vi "Run FGV Tests for String.vi"(2 "DELETE VI Reference":refnum<vi>, 3 "GET VI Reference":refnum<vi>, 4 "PUT VI Reference":refnum<vi>) -> (0 "Reason":string, 1 "Success":bool)   [LabVIEW 2013]
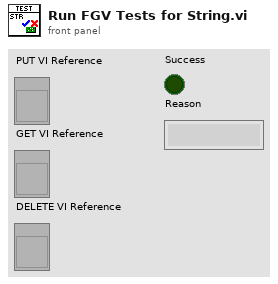
[diagram p1: front panel]
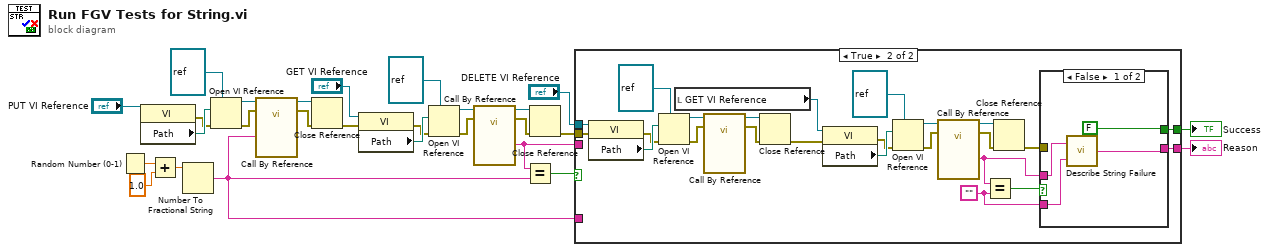
[diagram p0: block diagram]
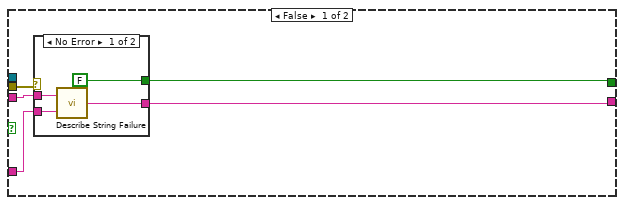
[diagram p2: hidden frame]
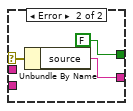
[diagram p3: hidden frame]
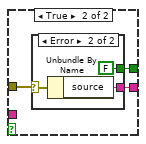
[diagram p4: hidden frame]
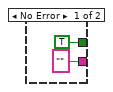
[diagram p5: hidden frame]
diagram:
  n1 = Random Number (0-1)() -> (number: 0 to 1=w12:dbl)
  n2 = property class="VI"(reference="PUT VI Reference") -> (error out=w5:errorcluster, "Path"=w18:path)  [unwired: 1 in, 1 out]
  n3 = Add(x=w12, y=1.0) -> (x+y=w2:dbl)
  n4 = Number To Fractional String(number=w2) -> (F-format string=w1:string)  [unwired: 3 in]
  n5 = Open VI Reference(type specifier VI Refnum (for type only)=refnum<vi> refnum, vi path=w18, error in (no error)=w5) -> (vi reference=w17:refnum<vi>, error out=w16:errorcluster)  [unwired: 3 in]
  n6 = call-by-ref "?"(reference=w17, error in=w16, "Division Input Channel"=w1) -> (reference out=w15:refnum<vi>, error out=w14:errorcluster)
  n7 = Close Reference(reference=w15, error in (no error)=w14) -> (error out=w10:errorcluster)
  n8 = property class="VI"(reference="GET VI Reference", error in=w10) -> (error out=w6:errorcluster, "Path"=w23:path)  [unwired: 1 out]
  n9 = Open VI Reference(type specifier VI Refnum (for type only)=refnum<vi> refnum, vi path=w23, error in (no error)=w6) -> (vi reference=w24:refnum<vi>, error out=w25:errorcluster)  [unwired: 3 in]
  n10 = call-by-ref "?"(reference=w24, error in=w25) -> (reference out=w26:refnum<vi>, error out=w27:errorcluster, "Division Input Channel"=w7:string)
  n11 = Equal?(x=w7, y=w1) -> (x = y?=w8:bool)
  n12 = Close Reference(reference=w26, error in (no error)=w27) -> (error out=w9:errorcluster)
  n13 = case shown="True" w8 {
    tunnel: "DELETE VI Reference" -> [_ w57]
    tunnel: w9 -> [w28 w56]
    tunnel: w1 -> [w31 _]
    tunnel: w7 -> [w32 _]
    tunnel: [w30 w42] -> w4
    tunnel: [w29 w41] -> w3
    frame False {
      n14 = case shown="No Error" w28 {
        selector: w28 -> [_ w39]
        tunnel: w32 -> [w36 _]
        tunnel: w31 -> [w35 _]
        tunnel: [FALSE FALSE] -> w30
        tunnel: [w33 w37] -> w29
        frame No Error {
          n15 = call "Describe String Failure.vi"("Expected"=w35, "Got"=w36) -> ("Failure Description"=w33:string)
        }
        frame Error {
          n16 = Unbundle By Name(w39) -> ("source"=w37:string)
        }
      }
    }
    frame True {
      w40 = ""
      n17 = property class="VI"(reference=w57, error in=w56) -> (error out=w46:errorcluster, "Path"=w59:path)  [unwired: 1 out]
      n18 = Open VI Reference(type specifier VI Refnum (for type only)=refnum<vi> refnum, vi path=w59, error in (no error)=w46) -> (vi reference=w60:refnum<vi>, error out=w61:errorcluster)  [unwired: 3 in]
      n19 = local read "GET VI Reference"() -> (w44:refnum<vi>)
      n20 = call-by-ref "?"(reference=w60, error in=w61) -> (reference out=w62:refnum<vi>, error out=w63:errorcluster)  [unwired: 1 in]
      n21 = Close Reference(reference=w62, error in (no error)=w63) -> (error out=w49:errorcluster)
      n22 = property class="VI"(reference=w44, error in=w49) -> (error out=w47:errorcluster, "Path"=w51:path)  [unwired: 1 out]
      n23 = Open VI Reference(type specifier VI Refnum (for type only)=refnum<vi> refnum, vi path=w51, error in (no error)=w47) -> (vi reference=w52:refnum<vi>, error out=w53:errorcluster)  [unwired: 3 in]
      n24 = call-by-ref "?"(reference=w52, error in=w53) -> (reference out=w54:refnum<vi>, error out=w55:errorcluster, "Division Input Channel"=w43:string)
      n25 = Equal?(x=w43, y=w40) -> (x = y?=w48:bool)
      n26 = Close Reference(reference=w54, error in (no error)=w55) -> (error out=w45:errorcluster)
      n27 = case shown="False" w48 {
        tunnel: w45 -> [_ w70]
        tunnel: w43 -> [w67 _]
        tunnel: w40 -> [w66 _]
        tunnel: [FALSE w69] -> w42
        tunnel: [w64 w68] -> w41
        frame False {
          n28 = call "Describe String Failure.vi"("Expected"=w66, "Got"=w67) -> ("Failure Description"=w64:string)
        }
        frame True {
          n29 = case shown="Error" w70 {
            selector: w70 -> [_ w75]
            tunnel: [TRUE FALSE] -> w69
            tunnel: ["" ("source") w73] -> w68
            frame No Error {
            }
            frame Error {
              n30 = Unbundle By Name(w75) -> ("source"=w73:string)
            }
          }
        }
      }
    }
  }
  "Success" <- w4
  "Reason" <- w3
